vi "Home.vi"(8 "error in (no error)":errorcluster, 11 "Stage_MadCityLabMicro in":refnum<class "Stage_MadCityLabMicro.lvclass">) -> (0 "error out":errorcluster, 3 "Stage_MadCityLabMicro out":refnum<class "Stage_MadCityLabMicro.lvclass">)   [LabVIEW 2020, in "Stage_MadCityLabMicro.lvlib" / "Stage_MadCityLabMicro.lvclass"]
uses:
  Stage_MadCityLabMicro.lvclass
  Stage_MadCityLabMicro.lvclass/Stage_MadCityLabMicro.ctl
  Hardware Abstraction Layer/Component/Device/Device/DataExchange.ctl
  Hardware Abstraction Layer/Component/Stage/Stage/Stage.lvclass
  Dependency/MicroDrive.dll
  Interface/DataListener/DataListener.lvclass
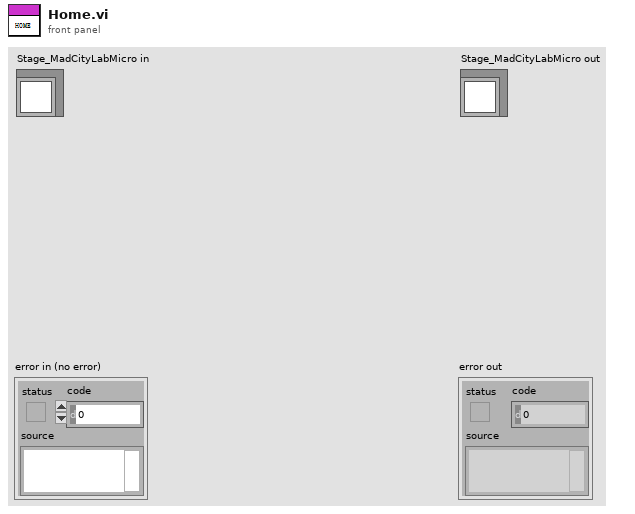
[diagram p1: front panel]
types:
  T1 = typedef "DataListener.lvclass/DataExchange.ctl" = cluster{"Source":string, "Destination":string, "Description":string, "value":variant}
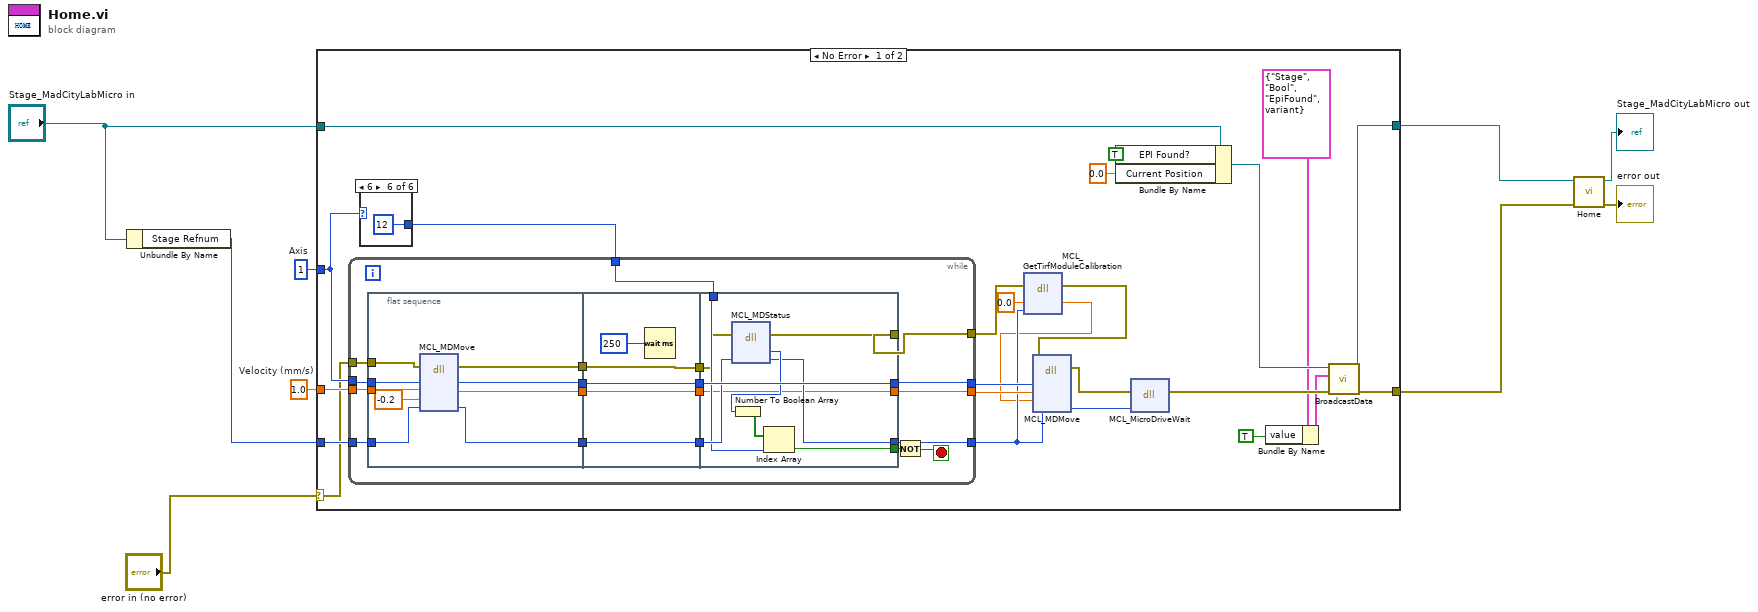
[diagram p0: block diagram]
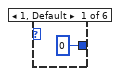
[diagram p2: hidden frame]
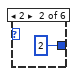
[diagram p3: hidden frame]
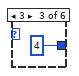
[diagram p4: hidden frame]
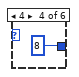
[diagram p5: hidden frame]
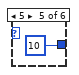
[diagram p6: hidden frame]
diagram:
  w5 = 1.0  # Velocity (mm/s)
  w6 = u16 1  # Axis
  n1 = Unbundle By Name("Stage_MadCityLabMicro in") -> ("Stage Refnum"=w7:i32)
  n2 = case shown="No Error" "error in (no error)" {
    selector: "error in (no error)" -> [w23 w84]
    tunnel: w5 -> [w33 _]
    tunnel: w7 -> [w32 _]
    tunnel: w6 -> [w29 _]
    tunnel: [w16 w84] -> w3
    tunnel: [w14 w83] -> w1
    tunnel: "Stage_MadCityLabMicro in" -> [w18 w83]
    frame No Error {
      n3 = case shown="6" w29 {
        tunnel: [0 2 4 8 10 12] -> w28
        frame 1, Default {
        }
        frame 2 {
        }
        frame 3 {
        }
        frame 4 {
        }
        frame 5 {
        }
        frame 6 {
        }
      }
      n4 = while {
        tunnel: w33 -> [w58]
        tunnel: w32 -> [w54]
        tunnel: [w53] -> w25
        tunnel: w29 -> [w56]
        tunnel: [w55] -> w31
        tunnel: w28 -> [w48]
        tunnel: [w44] -> w27
        tunnel: w23 -> [w43]
        tunnel: [w40] -> w22
        stop <- w57 stop-if-true
        n5 = flat-sequence {
          tunnel: w58 -> [w67]
          tunnel: w56 -> [w65]
          tunnel: w54 -> [w63]
          tunnel: [w64] -> w52
          tunnel: [w62] -> w51
          tunnel: [w61] -> w46
          tunnel: w43 -> [w60]
          tunnel: [w59] -> w42
          tunnel: w52 -> [w72]
          tunnel: w51 -> [w71]
          tunnel: [w72] -> w50
          tunnel: [w71] -> w49
          tunnel: w46 -> [w69]
          tunnel: [w69] -> w45
          tunnel: w42 -> [w68]
          tunnel: [w68] -> w41
          tunnel: [w78] -> w53
          tunnel: [w82] -> w55
          tunnel: w50 -> [w82]
          tunnel: w49 -> [w79]
          tunnel: w48 -> [w77]
          tunnel: [w76] -> w47
          tunnel: w45 -> [w75]
          tunnel: [w75] -> w44
          tunnel: w41 -> [w74]
          tunnel: [w73] -> w40
          frame #0 {
            n6 = dll-call lib="E:/Development/DevHardSoftware/MicroscopyFramework/Model/Hardware Layer/Real Hardware/Stage_MadCityLabMicro/Stage_MadCityLabMicro/Dependency/MicroDrive.dll" fn="MCL_MDMove"(error in=w60, "axis"=w65, "velocity"=w67, "distance"=-0.2, "handle"=w63) -> (error out=w59:errorcluster, "axis"=w64:i32, "velocity"=w61:dbl, "handle"=w62:i32)  [unwired: 3 in, 2 out]
          }
          frame #1 {
            n7 = Wait (ms)(milliseconds to wait=u32 250) -> ()  [unwired: 1 out]
          }
          frame #2 {
            n8 = dll-call lib="E:/Development/DevHardSoftware/MicroscopyFramework/Model/Hardware Layer/Real Hardware/Stage_MadCityLabMicro/Stage_MadCityLabMicro/Dependency/MicroDrive.dll" fn="MCL_MDStatus"(error in=w74, "handle"=w79) -> (error out=w73:errorcluster, "status"=w81:u16, "handle"=w78:i32)  [unwired: 2 in, 3 out]
            n9 = Number To Boolean Array(number=w81) -> (Boolean array=w80:bool[])
            n10 = Index Array(array=w80, index=w77) -> (element=w76:bool)
          }
        }
        n11 = Not(x=w47) -> (.not. x?=w57:bool)
      }
      n12 = dll-call lib="E:/Development/DevHardSoftware/MicroscopyFramework/Model/Hardware Layer/Real Hardware/Stage_MadCityLabMicro/Stage_MadCityLabMicro/Dependency/MicroDrive.dll" fn="MCL_GetTirfModuleCalibration"(error in=w22, "calMM"=0.0 ("distance"), "handle"=w25) -> (error out=w21:errorcluster, "calMM"=w24:dbl)  [unwired: 3 in, 2 out]
      n13 = dll-call lib="E:/Development/DevHardSoftware/MicroscopyFramework/Model/Hardware Layer/Real Hardware/Stage_MadCityLabMicro/Stage_MadCityLabMicro/Dependency/MicroDrive.dll" fn="MCL_MDMove"(error in=w21, "axis"=w31, "velocity"=w27, "distance"=w24, "handle"=w25) -> (error out=w20:errorcluster, "handle"=w30:i32)  [unwired: 4 in, 3 out]
      n14 = Bundle By Name(cluster=w18, "EPI Found?"=TRUE, "Current Position"=0.0) -> (w15:refnum<class "Stage_MadCityLabMicro.lvclass">)
      n15 = dll-call lib="E:/Development/DevHardSoftware/MicroscopyFramework/Model/Hardware Layer/Real Hardware/Stage_MadCityLabMicro/Stage_MadCityLabMicro/Dependency/MicroDrive.dll" fn="MCL_MicroDriveWait"(error in=w20, "handle"=w30) -> (error out=w19:errorcluster)  [unwired: 3 in, 2 out]
      n16 = Bundle By Name(cluster=T1 {"Source"="Stage", "Destination"="Bool", "Description"="EpiFound", "value"=variant} ("DataExchange"), "value"=TRUE) -> (w12:T1)
      n17 = call-dynamic "BroadcastData.vi"("error in (no error)"=w19, "DataExchange"=w12, "Device in"=w15) -> ("error out"=w16:errorcluster, "Device out"=w14:refnum<class "Stage_MadCityLabMicro.lvclass">)  [unwired: 7 in]
    }
    frame Error {
    }
  }
  n18 = call-parent "Home.vi"("error in (no error)"=w3, "Stage in"=w1) -> ("error out"=→"error out":errorcluster, "Stage out"=→"Stage_MadCityLabMicro out":refnum<class "Stage_MadCityLabMicro.lvclass">)  [unwired: 8 in]
